vi "cmd_status.vi"(3 "error in (no error)":errorcluster, 5 "HGF_SVMonitor":refnum<class "HGF_SVMonitor.lvclass">) -> (0 "error out":errorcluster, 1 "Registration Array":T1(array[cluster]), 2 "HGF_SVMonitor":refnum<class "HGF_SVMonitor.lvclass">)   [LabVIEW 2009]
doc: "Executes command \"status\"."
uses:
  HGF_SVMonitor.lvclass
  HGF_BaseClasses/HGF_NetworkVisitor/HGF_NetworkVisitor.lvclass
  HGF_BaseClasses/HGF_TriggeredEvent/HGF_TriggeredEvent.lvclass
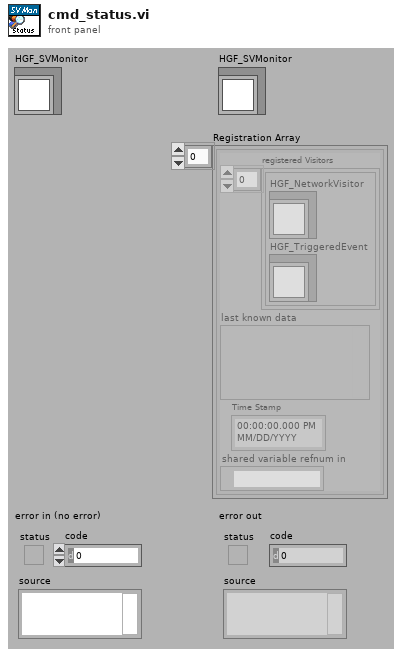
[diagram p1: front panel]
types:
  T1 = cluster{"registered Visitors":cluster{"HGF_NetworkVisitor":refnum<class "HGF_NetworkVisitor.lvclass">, "HGF_TriggeredEvent":refnum<class "HGF_TriggeredEvent.lvclass">}[], "last known data":variant, "Time Stamp":timestamp, "shared variable refnum in":refnum<k21>}[]
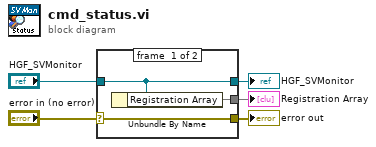
[diagram p0: block diagram]
diagram:
  n1 = case shown="No Error" "error in (no error)" {
    selector: "error in (no error)" -> [w8 w9]
    tunnel: [w8 w9] -> w4
    tunnel: [w7 w10] -> w2
    tunnel: "HGF_SVMonitor" -> [w7 w10]
    tunnel: [w6 _] -> w1
    frame #0 {
      n2 = Unbundle By Name(w7) -> ("Registration Array"=w6)
    }
    frame #1 {
    }
  }
  "error out" <- w4
  "HGF_SVMonitor" <- w2
  "Registration Array" <- w1
